vi "Create All Topologies.vi"() -> ()   [LabVIEW 2017]
uses:
  Slot Module Selection.ctl
panel:
  out "Status":string
  in  "Output Directory":path=path "C:/github/SLSC-Switch-Topology-Generator/output"
  in  "Source Base JSON File":path=path "C:/github/SLSC-Switch-Topology-Generator/source/json files/SET-2010 Base.json"
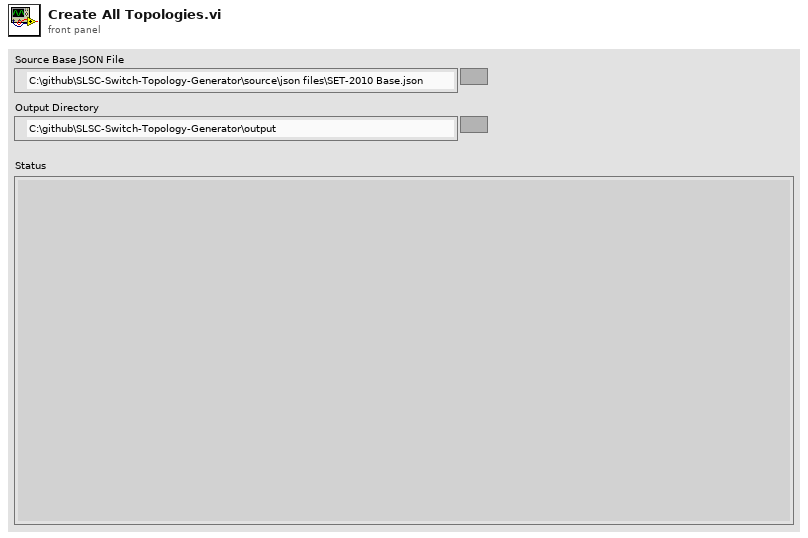
[diagram p1: front panel]
types:
  T1 = typedef "Slot Module Selection.ctl" = enum16{"Fault", "Instrument", "Empty"}
  T2 = cluster{"Slot 1 Module Selection":T1, "Slot 1 Module Selection 2":T1}[]
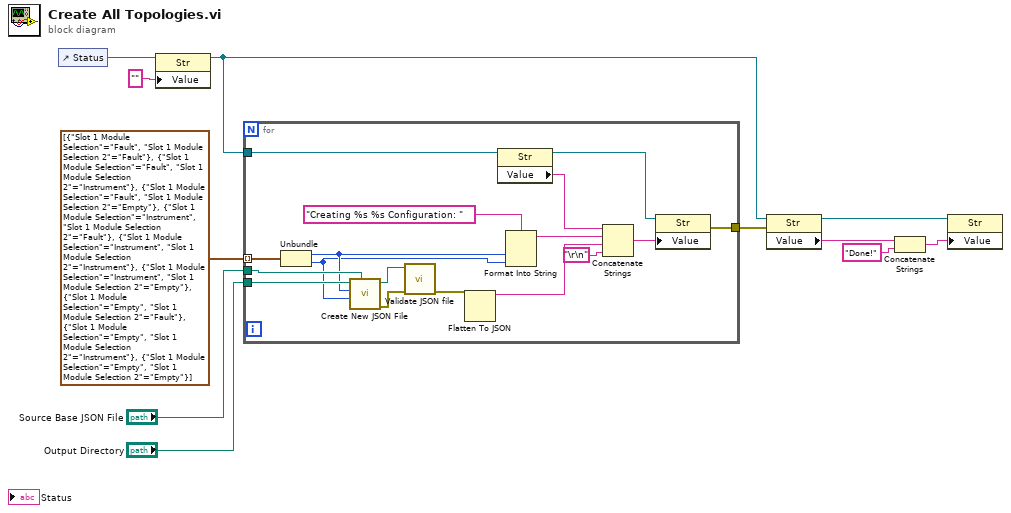
[diagram p0: block diagram]
diagram:
  n1 = control-ref of="Status"() -> (w4:refnum<vi>)
  n2 = property class="Str"(reference=w4, "Value"="") -> (reference out=w3:refnum<vi>)  [unwired: 1 in, 1 out]
  n3 = for {
    tunnel: "Source Base JSON File" -> [w28]
    tunnel: "Output Directory" -> [w27]
    tunnel: T2 [{"Slot 1 Module Selection"=enum."Fault", "Slot 1 Module Selection 2"=enum."Fault"}, {"Slot 1 Module Selection"=enum."Fault", "Slot 1 Module Selection 2"=enum."Instrument"}, {"Slot 1 Module Selection"=enum."Fault", "Slot 1 Module Selection 2"=enum."Empty"}, {"Slot 1 Module Selection"=enum."Instrument", "Slot 1 Module Selection 2"=enum."Fault"}, {"Slot 1 Module Selection"=enum."Instrument", "Slot 1 Module Selection 2"=enum."Instrument"}, {"Slot 1 Module Selection"=enum."Instrument", "Slot 1 Module Selection 2"=enum."Empty"}, {"Slot 1 Module Selection"=enum."Empty", "Slot 1 Module Selection 2"=enum."Fault"}, {"Slot 1 Module Selection"=enum."Empty", "Slot 1 Module Selection 2"=enum."Instrument"}, {"Slot 1 Module Selection"=enum."Empty", "Slot 1 Module Selection 2"=enum."Empty"}] -> [w26] mode=indexing
    tunnel: w3 -> [w25]
    tunnel: [w15] -> w1
    n4 = Unbundle(w26) -> ("Slot 1 Module Selection"=w24:T1, "Slot 1 Module Selection 2"=w23:T1)
    n5 = call "Create New JSON File.vi"("Source Base JSON File"=w28, "Slot 2 Module Selection"=w23, "Slot 1 Module Selection"=w24, "Output Directory"=w27) -> ("error out"=w14:errorcluster, "path out"=w13:path)  [unwired: 6 in]
    n6 = call "Validate JSON file.vi"("error in (no error)"=w14, "json file"=w13) -> ("error out"=w12:errorcluster)  [unwired: 9 in]
    n7 = Flatten To JSON(anything=w12) -> (JSON string=w19:string)  [unwired: 2 in, 1 out]
    n8 = property class="Str"(reference=w25) -> (reference out=w22:refnum<vi>, "Value"=w20:string)  [unwired: 1 in, 1 out]
    n9 = Format Into String(format string="Creating %s %s Configuration: ", w24, w23) -> (resulting string=w17:string)  [unwired: 2 in, 1 out]
    n10 = Concatenate Strings(w20, w17, w19, "\r\n") -> (w21:string)
    n11 = property class="Str"(reference=w22, "Value"=w21) -> (error out=w15:errorcluster)  [unwired: 1 in, 1 out]
  }
  n12 = property class="Str"(reference=w3, error in=w1) -> (reference out=w7:refnum<vi>, "Value"=w8:string)  [unwired: 1 out]
  n13 = Concatenate Strings(w8, "Done!" ("string")) -> (w6:string)
  n14 = property class="Str"(reference=w7, "Value"=w6) -> ()  [unwired: 1 in, 2 out]
